vi "Get PLC Type.vi"(9 "error in (no error)":errorcluster, 10 ".NET AdsDataType in":refnum<k24>) -> (1 "error out":errorcluster, 2 ".NET AdsDataType":refnum<k24>, 3 "PLC Type":T1)   [LabVIEW 2018, in "TwinCAT ADS.lvclass"]
uses:
  TwinCAT ADS.lvclass
  TwinCAT.Ads
  Controls/PLC Type.ctl
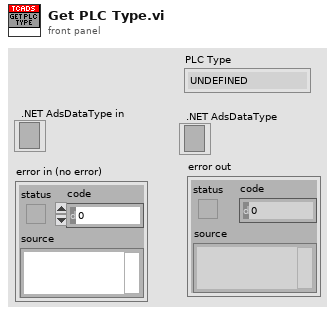
[diagram p1: front panel]
types:
  T1 = typedef "TwinCAT ADS.lvclass/PLC Type.ctl" = enum16{"UNDEFINED", "INT", "DINT", "REAL", "LREAL", "SINT", "BYTE", "UINT", "UDINT", "LINT", "ULINT", "STRING", "WSTRING", "BOOL", "TIME", "LTIME", "DATE", "DT", "TOD", "ARRAY", "JAGGED ARRAY", "STRUCT", "FUNCTION BLOCK", "UNION", "POINTER", "USER DEFINED"}
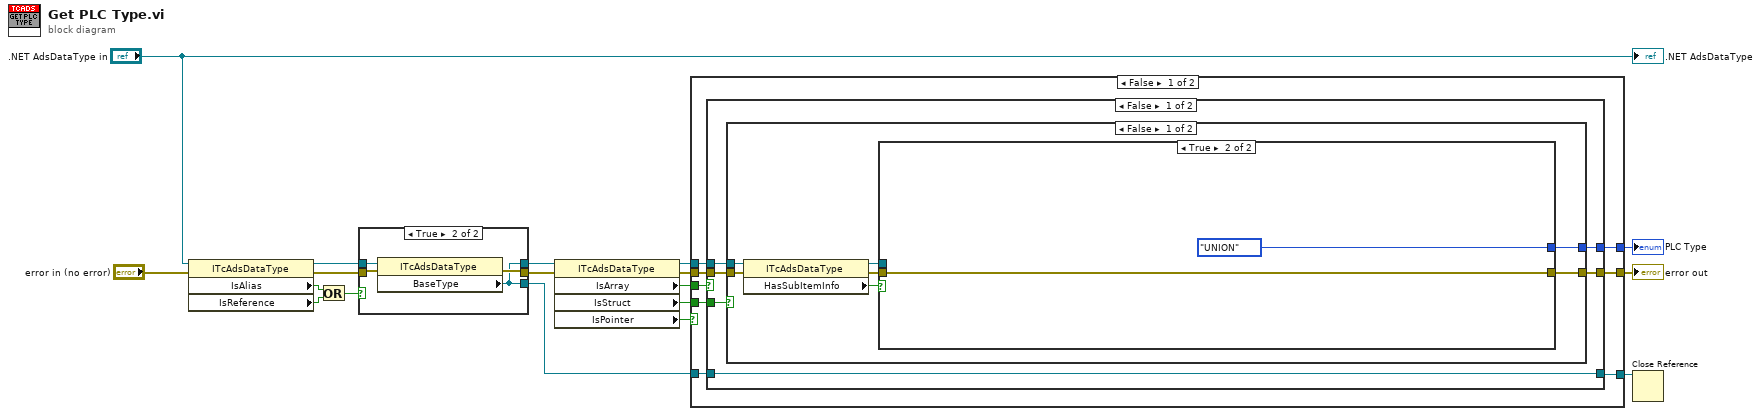
[diagram p0: block diagram]
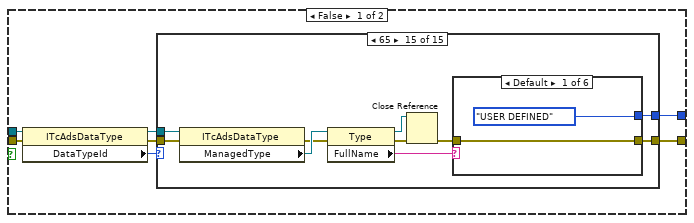
[diagram p3: hidden frame]
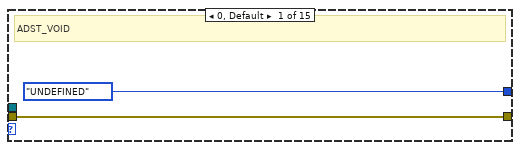
[diagram p4: hidden frame]
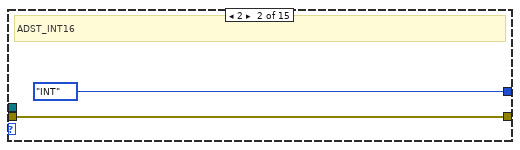
[diagram p5: hidden frame]
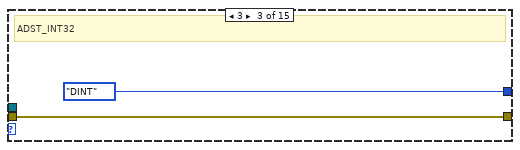
[diagram p6: hidden frame]
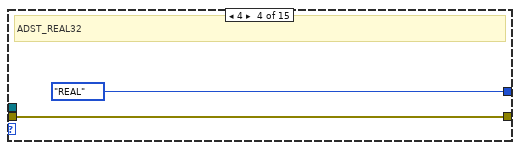
[diagram p7: hidden frame]
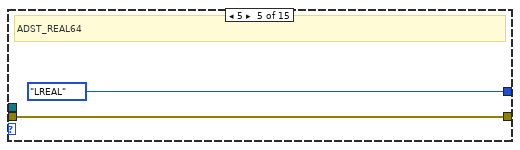
[diagram p8: hidden frame]
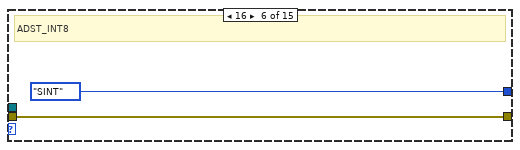
[diagram p9: hidden frame]
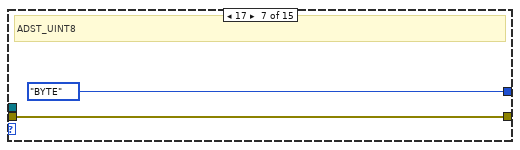
[diagram p10: hidden frame]
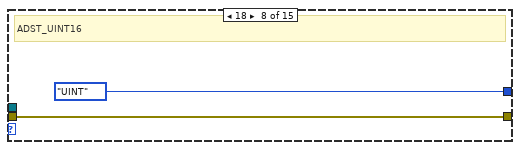
[diagram p11: hidden frame]
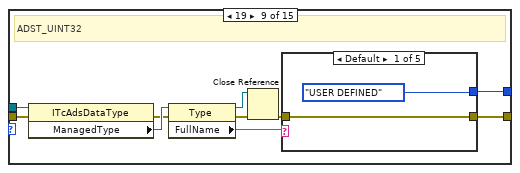
[diagram p12: hidden frame]
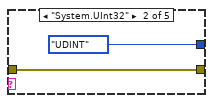
[diagram p13: hidden frame]
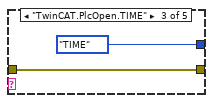
[diagram p14: hidden frame]
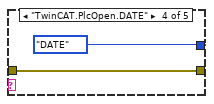
[diagram p15: hidden frame]
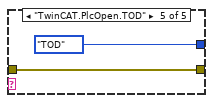
[diagram p16: hidden frame]
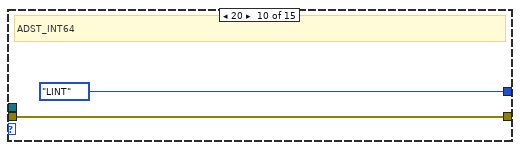
[diagram p17: hidden frame]
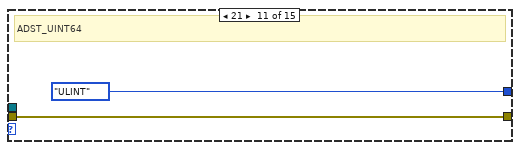
[diagram p18: hidden frame]
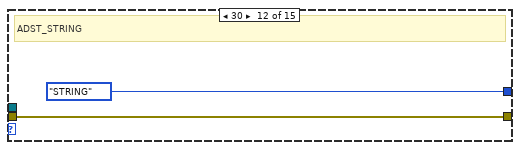
[diagram p19: hidden frame]
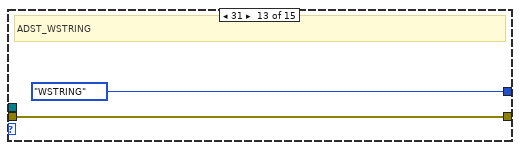
[diagram p20: hidden frame]
diagram:
  n1 = property class="ITcAdsDataType"(reference=".NET AdsDataType in", error in="error in (no error)") -> (reference out=w8:refnum<k24>, error out=w4:errorcluster, "IsAlias"=w6:bool, "IsReference"=w5:bool)
  n2 = Or(x=w6, y=w5) -> (x .or. y?=w7:bool)
  n3 = case shown="True" w7 {
    tunnel: w8 -> [w20 w24]
    tunnel: w4 -> [w19 w23]
    tunnel: [w20 w21] -> w3
    tunnel: [w19 w22] -> w2
    tunnel: [_ w21] -> w1
    frame False {
    }
    frame True {
      n4 = property class="ITcAdsDataType"(reference=w24, error in=w23) -> (error out=w22:errorcluster, "BaseType"=w21:refnum<k24>)  [unwired: 1 out]
    }
  }
  n5 = property class="ITcAdsDataType"(reference=w3, error in=w2) -> (reference out=w17:refnum<k24>, error out=w18:errorcluster, "IsArray"=w14:bool, "IsStruct"=w13:bool, "IsPointer"=w9:bool)
  n6 = case shown="False" w9 {
    tunnel: w18 -> [w32 w151]
    tunnel: w17 -> [w31 _]
    tunnel: [w30 PLC_Type."POINTER" ("PLC Type")] -> w16
    tunnel: [w29 w151] -> w15
    tunnel: w14 -> [w28 _]
    tunnel: w13 -> [w27 _]
    tunnel: w1 -> [w26 w152]
    tunnel: [w25 w152] -> w12
    frame False {
      n7 = case shown="False" w28 {
        tunnel: w32 -> [w38 w149]
        tunnel: w31 -> [w37 w148]
        tunnel: [w36 w145] -> w30
        tunnel: [w35 w147] -> w29
        tunnel: w27 -> [w34 _]
        tunnel: w26 -> [w33 w142]
        tunnel: [w33 w142] -> w25
        frame False {
          n8 = case shown="False" w34 {
            tunnel: w38 -> [w43 w135]
            tunnel: w37 -> [w42 w134]
            tunnel: [w45 w124] -> w36
            tunnel: [w44 w125] -> w35
            frame False {
              n9 = property class="ITcAdsDataType"(reference=w42, error in=w43) -> (reference out=w41:refnum<k24>, error out=w40:errorcluster, "HasSubItemInfo"=w39:bool)
              n10 = case shown="True" w39 {
                tunnel: [w52 PLC_Type."UNION" ("PLC Type")] -> w45
                tunnel: [w51 w122] -> w44
                tunnel: w41 -> [w49 _]
                tunnel: w40 -> [w50 w122]
                frame False {
                  n11 = property class="ITcAdsDataType"(reference=w49, error in=w50) -> (reference out=w47:refnum<k24>, error out=w48:errorcluster, "DataTypeId"=w46:i32)
                  n12 = case shown="65" w46 {
                    tunnel: [PLC_Type."UNDEFINED" ("PLC Type") PLC_Type."INT" ("PLC Type") PLC_Type."DINT" ("PLC Type") PLC_Type."REAL" ("PLC Type") PLC_Type."LREAL" ("PLC Type") PLC_Type."SINT" ("PLC Type") PLC_Type."BYTE" ("PLC Type") PLC_Type."UINT" ("PLC Type") w75 PLC_Type."LINT" ("PLC Type") PLC_Type."ULINT" ("PLC Type") PLC_Type."STRING" ("PLC Type") PLC_Type."WSTRING" ("PLC Type") PLC_Type."BOOL" ("PLC Type") w100] -> w52
                    tunnel: w48 -> [w54 w56 w58 w60 w62 w64 w66 w68 w71 w90 w92 w94 w95 w98 w105]
                    tunnel: [w54 w56 w58 w60 w62 w64 w66 w68 w78 w90 w92 w94 w95 w98 w99] -> w51
                    tunnel: w47 -> [_ _ _ _ _ _ _ _ w70 _ _ _ _ _ w104]
                    frame 0, Default {
                      # "ADST_VOID"
                    }
                    frame 2 {
                      # "ADST_INT16"
                    }
                    frame 3 {
                      # "ADST_INT32"
                    }
                    frame 4 {
                      # "ADST_REAL32"
                    }
                    frame 5 {
                      # "ADST_REAL64"
                    }
                    frame 16 {
                      # "ADST_INT8"
                    }
                    frame 17 {
                      # "ADST_UINT8"
                    }
                    frame 18 {
                      # "ADST_UINT16"
                    }
                    frame 19 {
                      # "ADST_UINT32"
                      n13 = property class="ITcAdsDataType"(reference=w70, error in=w71) -> (error out=w69:errorcluster, "ManagedType"=w77:refnum<k24>)  [unwired: 1 out]
                      n14 = property class="Type"(reference=w77, error in=w69) -> (reference out=w72:refnum<k24>, error out=w74:errorcluster, "FullName"=w76:string)
                      n15 = Close Reference(reference=w72, error in (no error)=w74) -> (error out=w73:errorcluster)
                      n16 = case shown="Default" w76 {
                        tunnel: [w80 w82 w84 w86 w88] -> w78
                        tunnel: w73 -> [w80 w82 w84 w86 w88]
                        tunnel: [PLC_Type."USER DEFINED" ("PLC Type") PLC_Type."UDINT" ("PLC Type") PLC_Type."TIME" ("PLC Type") PLC_Type."DATE" ("PLC Type") PLC_Type."TOD" ("PLC Type")] -> w75
                        frame Default {
                        }
                        frame "System.UInt32" {
                        }
                        frame "TwinCAT.PlcOpen.TIME" {
                        }
                        frame "TwinCAT.PlcOpen.DATE" {
                        }
                        frame "TwinCAT.PlcOpen.TOD" {
                        }
                      }
                    }
                    frame 20 {
                      # "ADST_INT64"
                    }
                    frame 21 {
                      # "ADST_UINT64"
                    }
                    frame 30 {
                      # "ADST_STRING"
                    }
                    frame 31 {
                      # "ADST_WSTRING"
                    }
                    frame 33 {
                      # "ADST_BIT"
                    }
                    frame 65 {
                      n17 = property class="ITcAdsDataType"(reference=w104, error in=w105) -> (error out=w103:errorcluster, "ManagedType"=w108:refnum<k24>)  [unwired: 1 out]
                      n18 = property class="Type"(reference=w108, error in=w103) -> (reference out=w106:refnum<k24>, error out=w107:errorcluster, "FullName"=w102:string)
                      n19 = Close Reference(reference=w106, error in (no error)=w107) -> (error out=w101:errorcluster)
                      n20 = case shown="Default" w102 {
                        tunnel: [w110 w112 w114 w116 w118 w120] -> w99
                        tunnel: w101 -> [w110 w112 w114 w116 w118 w120]
                        tunnel: [PLC_Type."USER DEFINED" ("PLC Type") PLC_Type."TIME" ("PLC Type") PLC_Type."LTIME" ("PLC Type") PLC_Type."DATE" ("PLC Type") PLC_Type."DT" ("PLC Type") PLC_Type."TOD" ("PLC Type")] -> w100
                        frame Default {
                        }
                        frame "TwinCAT.PlcOpen.TIME" {
                        }
                        frame "TwinCAT.PlcOpen.LTIME" {
                        }
                        frame "TwinCAT.PlcOpen.DATE" {
                        }
                        frame "TwinCAT.PlcOpen.DT" {
                        }
                        frame "TwinCAT.PlcOpen.TOD" {
                        }
                      }
                    }
                  }
                }
                frame True {
                }
              }
            }
            frame True {
              n21 = property class="ITcAdsDataType"(reference=w134, error in=w135) -> (error out=w133:errorcluster, "SubItems"=w132:refnum<k24>)  [unwired: 1 out]
              n22 = invoke class="ReadOnlySubItemCollection" method="get_Item"(reference=w132, error in=w133, "index"=0) -> (reference out=w128:refnum<k24>, error out=w130:errorcluster, "get_Item"=w129:refnum<k24>)  [unwired: 1 in, 1 out]
              n23 = Close Reference(reference=w128) -> ()  [unwired: 1 in, 1 out]
              n24 = property class="ITcAdsSubItem"(reference=w129, error in=w130) -> (reference out=w123:refnum<k24>, error out=w126:errorcluster, "Offset"=w127:i32)
              n25 = Close Reference(reference=w123) -> ()  [unwired: 1 in, 1 out]
              n26 = case shown="0" w127 {
                tunnel: w126 -> [w137 w139 w141]
                tunnel: [w137 w139 w141] -> w125
                tunnel: [PLC_Type."UNDEFINED" ("PLC Type") PLC_Type."STRUCT" ("PLC Type") PLC_Type."FUNCTION BLOCK" ("PLC Type")] -> w124
                frame ..-1 {
                }
                frame 0 {
                }
                frame 1.. {
                }
              }
            }
          }
        }
        frame True {
          n27 = property class="ITcAdsDataType"(reference=w148, error in=w149) -> (error out=w147:errorcluster, "IsJaggedArray"=w146:bool)  [unwired: 1 out]
          n28 = Select(t=PLC_Type."JAGGED ARRAY" ("PLC Type"), s=w146, f=PLC_Type."ARRAY" ("PLC Type")) -> (s? t:f=w145:T1)
        }
      }
    }
    frame True {
    }
  }
  "error out" <- w15
  "PLC Type" <- w16
  n29 = Close Reference(reference=w12) -> ()  [unwired: 1 in, 1 out]
  ".NET AdsDataType" <- ".NET AdsDataType in"
